vi "Get Selected DAQChannel.vi"(8 "error in (no error)":errorcluster, 11 "UI in":refnum<class "UI.lvclass">) -> (0 "error out":errorcluster, 1 "Type":enum16{"AO", "DO", "AI"}(ring), 2 "Channel Out":tag, 3 "UI out":refnum<class "UI.lvclass">)   [LabVIEW 2015, in "UI.lvlib" / "UI.lvclass"]
uses:
  UI.lvclass
  UI.lvclass/UI.ctl
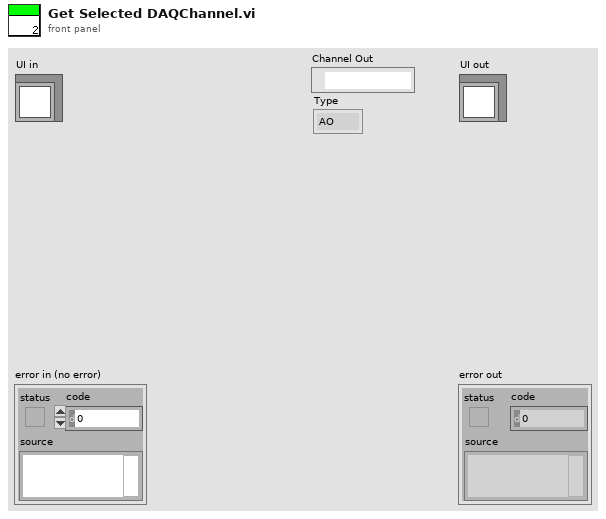
[diagram p1: front panel]
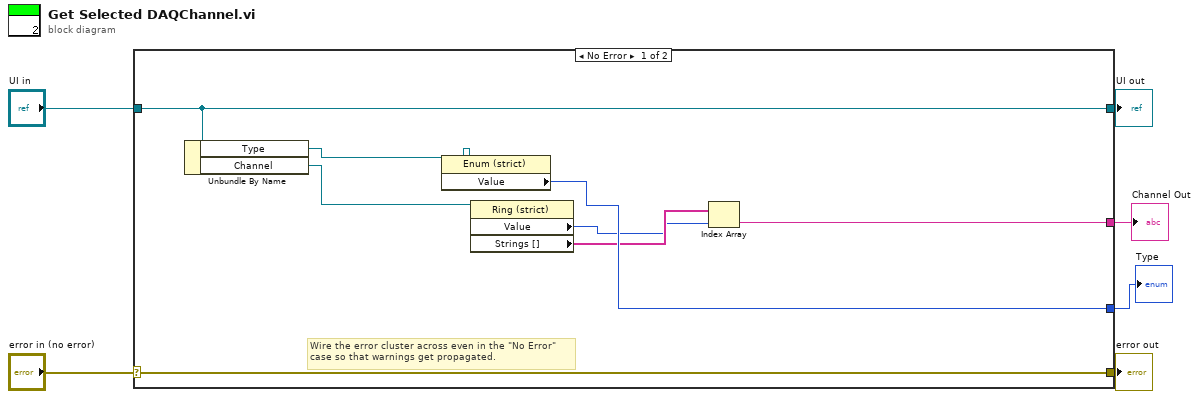
[diagram p0: block diagram]
diagram:
  n1 = case shown="No Error" "error in (no error)" {
    selector: "error in (no error)" -> [w14 w16]
    tunnel: [w14 w16] -> w5
    tunnel: [w11 w15] -> w3
    tunnel: "UI in" -> [w11 w15]
    tunnel: [w7 _] -> w2
    tunnel: [w10 _] -> w1
    frame No Error {
      # "Wire the error cluster across even in the \"No Error\"\ncase so that warnings get propagated."
      n2 = Unbundle By Name(w11) -> ("Type"=w13:refnum<vi>, "Channel"=w12:refnum<vi>)
      n3 = property class="Enum (strict)"(reference=w13) -> ("Value"=w10:enum16{"AO", "DO", "AI"})  [unwired: 1 in, 2 out]
      n4 = property class="Ring (strict)"(reference=w12) -> ("Value"=w8:u16, "Strings []"=w9:string[])  [unwired: 1 in, 2 out]
      n5 = Index Array(array=w9, index=w8) -> (element=w7:string)
    }
    frame Error {
    }
  }
  "error out" <- w5
  "UI out" <- w3
  "Channel Out" <- w2
  "Type" <- w1
